vi "Compute Convex Hull.vi"(8 "error in (no error)":errorcluster, 11 "Video Cam Processor in":refnum<class "Video Cam Processor.lvclass">) -> (0 "error out":errorcluster, 3 "Video Cam Processor out":refnum<class "Video Cam Processor.lvclass">)   [LabVIEW 2018, in "Video Cam Processor.lvclass"]
uses:
  Video Cam Processor.lvclass
  Video Cam Processor.lvclass/Video Cam Processor.ctl
  44cf60d7-18dc-4b7f-9b2d-e99ad05a6dbc.vi
  44cf60d7-18dc-4b7f-9b2d-e99ad05a6dbc.vi/853abcf9-27cb-4907-8391-14211514108e.vi
panel:
  out "Complete":dbl(slide) scale=0.0..1.0
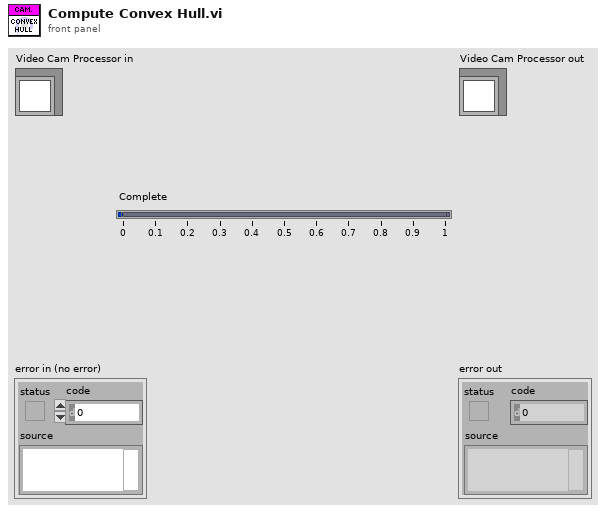
[diagram p1: front panel]
types:
  T1 = typedef "IMAQ Image.ctl" = refnum<image>
  T2 = cluster{"Area":dbl, "Number of Holes":dbl, "Bounding Rect":cluster{"Left":dbl, "Top":dbl, "Right":dbl, "Bottom":dbl}, "Center of Mass":cluster{"X":dbl, "Y":dbl}, "Orientation":dbl, "Dimensions":cluster{"Width":dbl, "Height":dbl}}[]
  T3 = typedef "Graham Scan Point.ctl" = cluster{"X":i32, "Y":i32}
  T4 = typedef "Video Cam Processor.lvclass/Hull Point STYP.ctl" = cluster{"X":i32, "Y":i32}
  T5 = cluster{"Area":dbl, "Number of Holes":dbl, "Bounding Rect":cluster{"Left":dbl, "Top":dbl, "Right":dbl, "Bottom":dbl}, "Center of Mass":cluster{"X":dbl, "Y":dbl}, "Orientation":dbl, "Dimensions":cluster{"Width":dbl, "Height":dbl}}
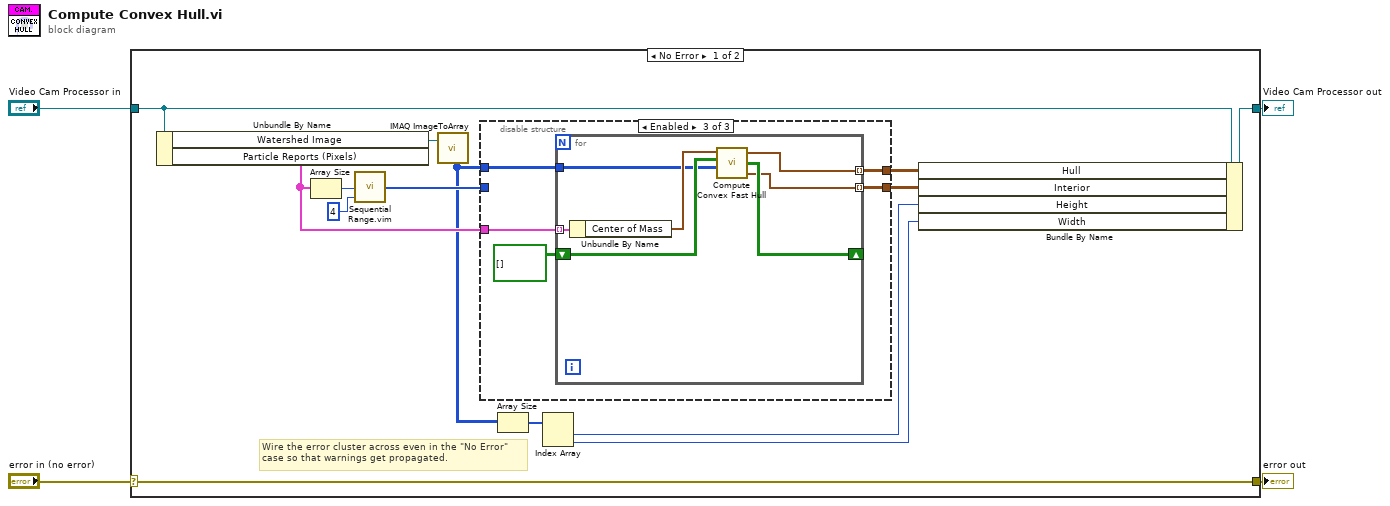
[diagram p0: block diagram]
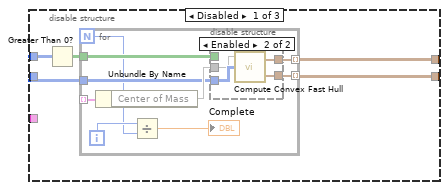
[diagram p2: hidden frame]
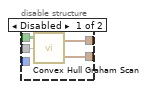
[diagram p3: hidden frame]
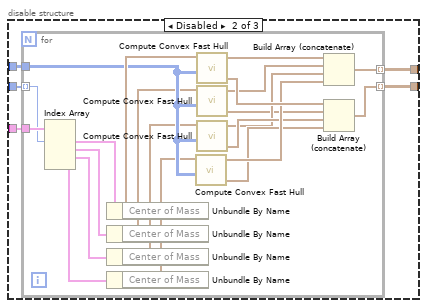
[diagram p4: hidden frame]
diagram:
  n1 = case shown="No Error" "error in (no error)" {
    selector: "error in (no error)" -> [w18 w79]
    tunnel: [w18 w79] -> w3
    tunnel: [w13 w78] -> w1
    tunnel: "Video Cam Processor in" -> [w16 w78]
    frame No Error {
      # "Wire the error cluster across even in the \"No Error\"\ncase so that warnings get propagated."
      n2 = Unbundle By Name(w16) -> ("Watershed Image"=w17:T1, "Particle Reports (Pixels)"=w9:T2)
      n3 = Array Size(array=w9) -> (size(s)=w12:i32)
      n4 = call "Sequential Range.vim"("Increment (1)"=4, "Stop (exc.)"=w12) -> ("Range(st, stp, inc)"=w10:i32[])  [unwired: 1 in]
      n5 = call "IMAQ ImageToArray"("Image"=w17) -> ("Image Pixels (U16)"=w8:u16[][])  [unwired: 3 in, 4 out]
      n6 = disable-structure shown="Enabled" {
        disable-tunnel: [w21 w40 w68] -> w15
        disable-tunnel: [w20 w41 w67] -> w14
        disable-tunnel: w8 -> [w19 w44 w69]
        disable-tunnel: w10 -> [_ w43 _]
        disable-tunnel: w9 -> [_ w42 w70]
        frame Disabled {
          n7 = Greater Than 0?(x=w19) -> (x > 0?=w22:bool[][])
          n8 = for {
            N -> [w24]
            tunnel: w22 -> [w29]
            tunnel: _ -> [w31] mode=indexing
            tunnel: [w28] -> w21 mode=indexing
            tunnel: [w27] -> w20 mode=indexing
            tunnel: w19 -> [w26]
            i -> [w25]
            n9 = Unbundle By Name(w31) -> ("Center of Mass"=w30)
            n10 = Divide(x=w25, y=w24) -> (x/y=→"Complete":dbl)
            n11 = disable-structure shown="Enabled" {
              disable-tunnel: w30 -> [w35 w36]
              disable-tunnel: w29 -> [w34 _]
              disable-tunnel: [w33 w38] -> w28
              disable-tunnel: [w32 w37] -> w27
              disable-tunnel: w26 -> [_ w39]
              frame Disabled {
                n12 = call "Convex Hull Graham Scan.vi"("Bounding Rectangle (Entire Array)"=w35, "Plane"=w34) -> ("Interior Points"=w32:T3[], "Convex Hull"=w33:T3[])  [unwired: 1 in]
              }
              frame Enabled {
                n13 = call "Compute Convex Fast Hull.vi"("Data"=w39, "Center of Mass (0, 0)"=w36) -> ("Interior"=w37:T4[], "Hull"=w38:T4[])  [unwired: 1 in]
              }
            }
          }
        }
        frame Disabled {
          n14 = for {
            tunnel: w44 -> [w54]
            tunnel: w43 -> [w64] mode=indexing
            tunnel: w42 -> [w65]
            tunnel: [w59] -> w41 mode=indexing
            tunnel: [w58] -> w40 mode=indexing
            n15 = Index Array(array=w65, index #1=w64) -> (element #1=w63:T5, element #2=w62:T5, element #3=w61:T5, element #4=w60:T5)  [unwired: 3 in]
            n16 = Unbundle By Name(w63) -> ("Center of Mass"=w57:cluster{"X":dbl, "Y":dbl})
            n17 = Unbundle By Name(w62) -> ("Center of Mass"=w45:cluster{"X":dbl, "Y":dbl})
            n18 = Unbundle By Name(w61) -> ("Center of Mass"=w48:cluster{"X":dbl, "Y":dbl})
            n19 = Unbundle By Name(w60) -> ("Center of Mass"=w53:cluster{"X":dbl, "Y":dbl})
            n20 = call "Compute Convex Fast Hull.vi"("Data"=w54, "Center of Mass (0, 0)"=w53) -> ("Interior"=w51:T4[], "Hull"=w52:T4[])  [unwired: 2 in, 1 out]
            n21 = call "Compute Convex Fast Hull.vi"("Data"=w54, "Center of Mass (0, 0)"=w57) -> ("Interior"=w55:T4[], "Hull"=w56:T4[])  [unwired: 2 in, 1 out]
            n22 = call "Compute Convex Fast Hull.vi"("Data"=w54, "Center of Mass (0, 0)"=w45) -> ("Interior"=w47:T4[], "Hull"=w46:T4[])  [unwired: 2 in, 1 out]
            n23 = call "Compute Convex Fast Hull.vi"("Data"=w54, "Center of Mass (0, 0)"=w48) -> ("Interior"=w50:T4[], "Hull"=w49:T4[])  [unwired: 2 in, 1 out]
            n24 = Build Array (concatenate)(w56, w46, w49, w52) -> (w58:T4[])
            n25 = Build Array (concatenate)(w55, w47, w50, w51) -> (w59:T4[])
          }
        }
        frame Enabled {
          n26 = for {
            tunnel: w70 -> [w77] mode=indexing
            tunnel: w69 -> [w73]
            shift-right: [w75] -> _
            shift-left: bool[][] [] ("Visited Out") -> [w74]
            tunnel: [w72] -> w68 mode=indexing
            tunnel: [w71] -> w67 mode=indexing
            n27 = Unbundle By Name(w77) -> ("Center of Mass"=w76:cluster{"X":dbl, "Y":dbl})
            n28 = call "Compute Convex Fast Hull.vi"("Data"=w73, "Visited"=w74, "Center of Mass (0, 0)"=w76) -> ("Interior"=w71:T4[], "Visited Out"=w75:bool[][], "Hull"=w72:T4[])  [unwired: 1 in]
          }
        }
      }
      n29 = Array Size(array=w8) -> (size(s)=w7:i32[])
      n30 = Index Array(array=w7) -> (element #1=w6:i32, element #2=w5:i32)  [unwired: 2 in]
      n31 = Bundle By Name(cluster=w16, "Hull"=w15, "Interior"=w14, "Height"=w6, "Width"=w5) -> (w13:refnum<class "Video Cam Processor.lvclass">)
    }
    frame Error {
    }
  }
  "error out" <- w3
  "Video Cam Processor out" <- w1
